vi "HolDrvCtrl_PackPID.vi"(8 "Period":dbl=0.02, 10 "Y PID Tuning":T1={"Kp"=0.0, "Ki"=0.0, "Kd"=0.0, "MaximumIntegral"=9.9e+30, "MinimumIntegral"=-9.9e+30}, 11 "X PID Tuning":T1={"Kp"=0.0, "Ki"=0.0, "Kd"=0.0, "MaximumIntegral"=9.9e+30, "MinimumIntegral"=-9.9e+30}) -> (2 "Y PID CONTROLLER":T2={"Kp"=0.0, "Ki"=0.0, "Kd"=0.0, "Period"=0.0, "Max_Integral"=0.0, "Min_Integral"=0.0, "Max_Input"=0.0, "Min_Input"=0.0, "Continuous"=FALSE, "PositionError"=0.0, "VelocityError"=0.0, "PrevError"=0.0, "TotalError"=0.0, "PositionTolerance"=0.0, "VelocityTolerance"=0.0, "SetPoint"=0.0, "Kf"=0.0, "Prev_Deriv"=0.0, "Prev_Deriv 2"=0.0, "DerivativeFilter"=FALSE, "Min_Output"=-9.99e+35, "Max_Output"=9.9e+35, "Prev_F_P"=0.0, "Prev_F_P_2"=0.0, "AntiWindupActive"=FALSE, "Measurement"=0.0} {"Measurement" format="%16_6e"; "Prev_F_P_2" format="%16_6e"; "Prev_F_P" format="%16_6e"; "Max_Output" format="%16_6e"; "Min_Output" format="%16_6e"; "Prev_Deriv 2" format="%16_6e"; "Prev_Deriv" format="%16_6e"; "Kf" format="%16_6e"; "SetPoint" format="%16_6e"; "VelocityTolerance" format="%16_6e"; "PositionTolerance" format="%16_6e"; "TotalError" format="%16_6e"; "PrevError" format="%16_6e"; "VelocityError" format="%16_6e"; "PositionError" format="%16_6e"; "Min_Input" format="%16_6e"; "Max_Input" format="%16_6e"; "Min_Integral" format="%16_6e"; "Max_Integral" format="%16_6e"; "Period" format="%16_6e"; "Kd" format="%16_6e"; "Ki" format="%16_6e"; "Kp" format="%16_6e"}, 3 "X PID_CONTROLLER":T2={"Kp"=0.0, "Ki"=0.0, "Kd"=0.0, "Period"=0.0, "Max_Integral"=0.0, "Min_Integral"=0.0, "Max_Input"=0.0, "Min_Input"=0.0, "Continuous"=FALSE, "PositionError"=0.0, "VelocityError"=0.0, "PrevError"=0.0, "TotalError"=0.0, "PositionTolerance"=0.0, "VelocityTolerance"=0.0, "SetPoint"=0.0, "Kf"=0.0, "Prev_Deriv"=0.0, "Prev_Deriv 2"=0.0, "DerivativeFilter"=FALSE, "Min_Output"=-9.99e+35, "Max_Output"=9.9e+35, "Prev_F_P"=0.0, "Prev_F_P_2"=0.0, "AntiWindupActive"=FALSE, "Measurement"=0.0} {"Measurement" format="%16_6e"; "Prev_F_P_2" format="%16_6e"; "Prev_F_P" format="%16_6e"; "Max_Output" format="%16_6e"; "Min_Output" format="%16_6e"; "Prev_Deriv 2" format="%16_6e"; "Prev_Deriv" format="%16_6e"; "Kf" format="%16_6e"; "SetPoint" format="%16_6e"; "VelocityTolerance" format="%16_6e"; "PositionTolerance" format="%16_6e"; "TotalError" format="%16_6e"; "PrevError" format="%16_6e"; "VelocityError" format="%16_6e"; "PositionError" format="%16_6e"; "Min_Input" format="%16_6e"; "Max_Input" format="%16_6e"; "Min_Integral" format="%16_6e"; "Max_Integral" format="%16_6e"; "Period" format="%16_6e"; "Kd" format="%16_6e"; "Ki" format="%16_6e"; "Kp" format="%16_6e"})   [LabVIEW 2019, in "Trajectory_Library.lvlib"]
doc: "Convience, single call, LabVIEW function. Packs \"standard\" constants for the X and Y PID controllers used by the holonomic controller. \n\nNOTE -- This version does NOT support dynamic tuning. The constants are read only used during the first execution cycle.\n \nInputs:\n - X PID Tuning -- PID Tuning parameters containing:\n - Kp -- The proportional coefficient.\n - Ki -- The integral coefficient.\n - Kd -- The derivative coefficient.\n - Maximum Integral -- The maximum value of the integrator.\n - Minimum Integral -- The minimum value of the integrator.\n - Y PID Tuning -- PID Tuning parameters containing:\n - Kp -- The proportional coefficient.\n - Ki -- The integral coefficient.\n - Kd -- The derivative coefficient.\n - Maximum Integral -- The maximum value of the integrator.\n - Minimum Integral -- The minimum value of the integrator.\n - Period -- Period of repeated calls in seconds. (Default: 0.020)\n\n\nOutputs:\n - X PID_Controller -- Created X PID_Controller data cluster\n - Y PID_Controller -- Created Y PID_Controller data cluster"
uses:
  Trajectory_Library.lvlib
  TypeDef/PID_CONTROLLER.ctl
  TypeDef/PID_TUNING.ctl
  <vilib>/Rock Robotics/SystemInterfaces/NetworkCommunication/NetComm_UsageReport_report.vi
  Globals/Util_LibraryGlobals.vi
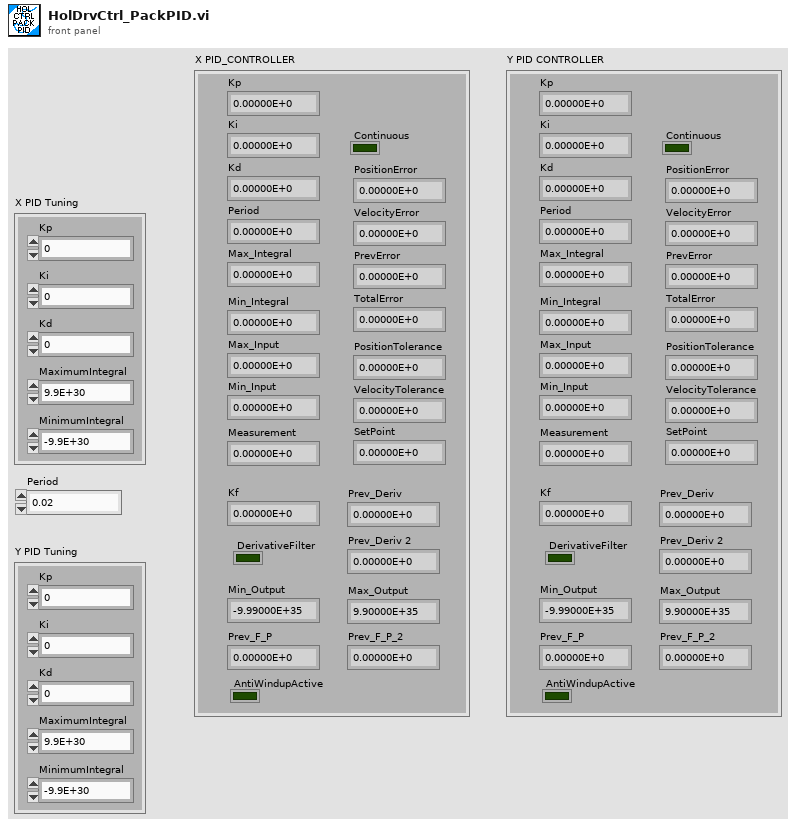
[diagram p1: front panel]
types:
  T1 = typedef "Trajectory_Library.lvlib/PID_TUNING.ctl" = cluster{"Kp":dbl, "Ki":dbl, "Kd":dbl, "MaximumIntegral":dbl, "MinimumIntegral":dbl}
  T2 = typedef "Trajectory_Library.lvlib/PID_CONTROLLER.ctl" = cluster{"Kp":dbl, "Ki":dbl, "Kd":dbl, "Period":dbl, "Max_Integral":dbl, "Min_Integral":dbl, "Max_Input":dbl, "Min_Input":dbl, "Continuous":bool, "PositionError":dbl, "VelocityError":dbl, "PrevError":dbl, "TotalError":dbl, "PositionTolerance":dbl, "VelocityTolerance":dbl, "SetPoint":dbl, "Kf":dbl, "Prev_Deriv":dbl, "Prev_Deriv 2":dbl, "DerivativeFilter":bool, "Min_Output":dbl, "Max_Output":dbl, "Prev_F_P":dbl, "Prev_F_P_2":dbl, "AntiWindupActive":bool, "Measurement":dbl}
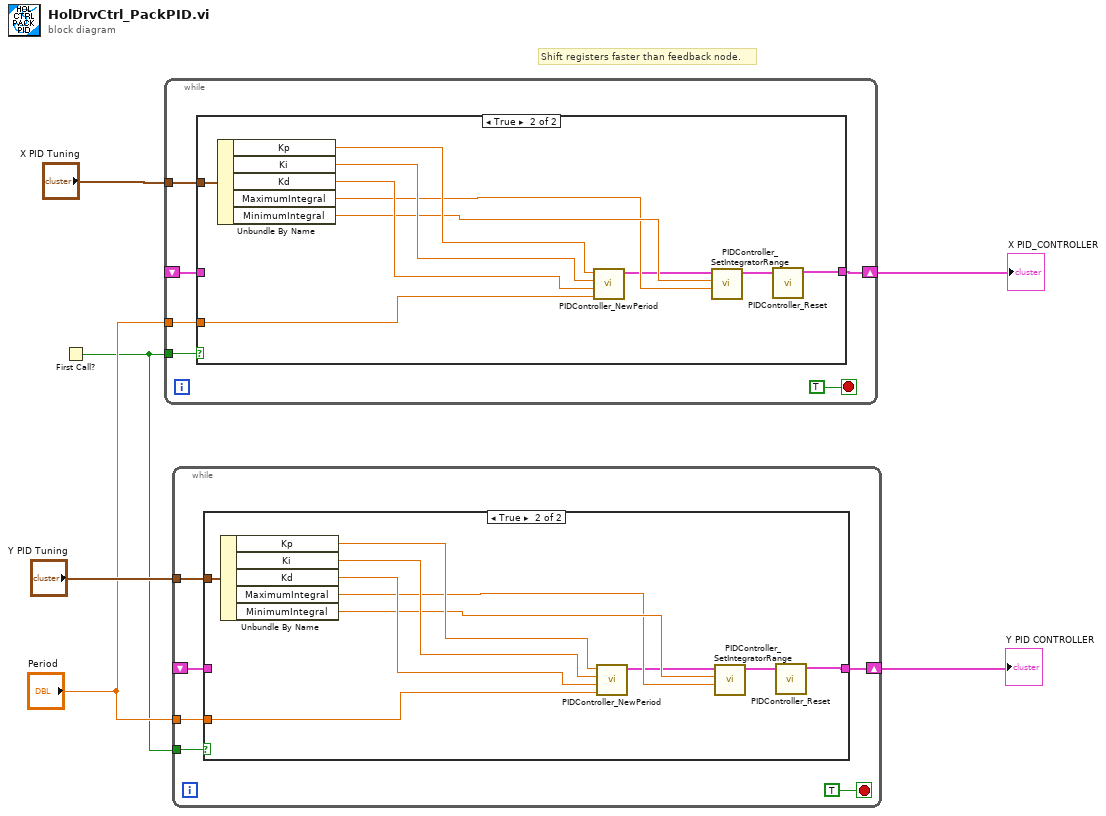
[diagram p0: block diagram]
diagram:
  # "Shift registers faster than feedback node."
  n1 = First Call?() -> (First Call?: T/F=w2:bool)
  n2 = while {
    tunnel: "X PID Tuning" -> [w12]
    tunnel: "Period" -> [w10]
    tunnel: w2 -> [w9]
    shift-right: [w11] -> w1
    shift-left: _ -> [w7]
    stop <- TRUE stop-if-true
    n3 = case shown="True" w9 {
      tunnel: w12 -> [_ w23]
      tunnel: [w13 w17] -> w11
      tunnel: w10 -> [_ w14]
      tunnel: w7 -> [w13 _]
      frame False {
      }
      frame True {
        n4 = Unbundle By Name(w23) -> ("Kp"=w22:dbl, "Ki"=w20:dbl, "Kd"=w21:dbl, "MaximumIntegral"=w18:dbl, "MinimumIntegral"=w19:dbl)
        n5 = call "PIDController_NewPeriod.vi"("Period"=w14, "Kd"=w21, "Ki"=w20, "Kp"=w22) -> ("PID_CONTROLLER"=w16:T2)  [unwired: 7 in]
        n6 = call "PIDController_SetIntegratorRange.vi"("MaximumIntegral"=w18, "MinimumIntegral"=w19, "in PID_CONTROLLER"=w16) -> ("out PID_CONTROLLER"=w15:T2)  [unwired: 8 in]
        n7 = call "PIDController_Reset.vi"("in PID_CONTROLLER"=w15) -> ("out PID_CONTROLLER"=w17:T2)  [unwired: 10 in]
      }
    }
  }
  "X PID_CONTROLLER" <- w1
  n8 = while {
    tunnel: "Y PID Tuning" -> [w28]
    tunnel: "Period" -> [w27]
    tunnel: w2 -> [w26]
    shift-right: [w29] -> w5
    shift-left: _ -> [w24]
    stop <- TRUE stop-if-true
    n9 = case shown="True" w26 {
      tunnel: w28 -> [_ w40]
      tunnel: [w30 w34] -> w29
      tunnel: w27 -> [_ w31]
      tunnel: w24 -> [w30 _]
      frame False {
      }
      frame True {
        n10 = Unbundle By Name(w40) -> ("Kp"=w39:dbl, "Ki"=w37:dbl, "Kd"=w38:dbl, "MaximumIntegral"=w35:dbl, "MinimumIntegral"=w36:dbl)
        n11 = call "PIDController_NewPeriod.vi"("Period"=w31, "Kd"=w38, "Ki"=w37, "Kp"=w39) -> ("PID_CONTROLLER"=w33:T2)  [unwired: 7 in]
        n12 = call "PIDController_SetIntegratorRange.vi"("MaximumIntegral"=w35, "MinimumIntegral"=w36, "in PID_CONTROLLER"=w33) -> ("out PID_CONTROLLER"=w32:T2)  [unwired: 8 in]
        n13 = call "PIDController_Reset.vi"("in PID_CONTROLLER"=w32) -> ("out PID_CONTROLLER"=w34:T2)  [unwired: 10 in]
      }
    }
  }
  "Y PID CONTROLLER" <- w5
